vi "ORS_AlazarDLLAcq_Start.vi"(8 "error in (no error)":errorcluster, 11 "ATSHandle":u32) -> (0 "error out":errorcluster, 3 "ATSHandle_out":u32)   [LabVIEW 2024]
panel:
  out "path out":path
  out "return code":i32
  out "dt":u32=26
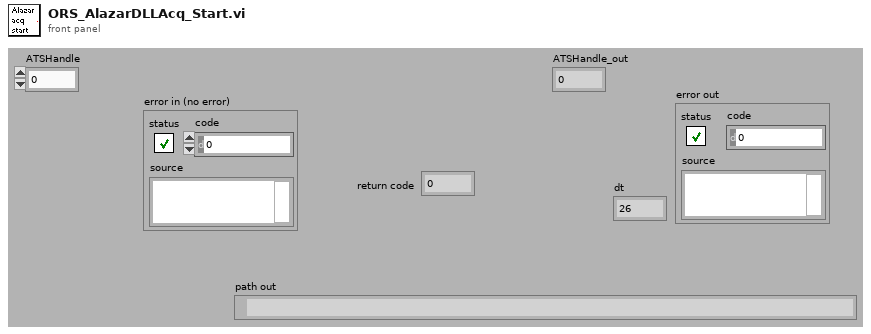
[diagram p1: front panel]
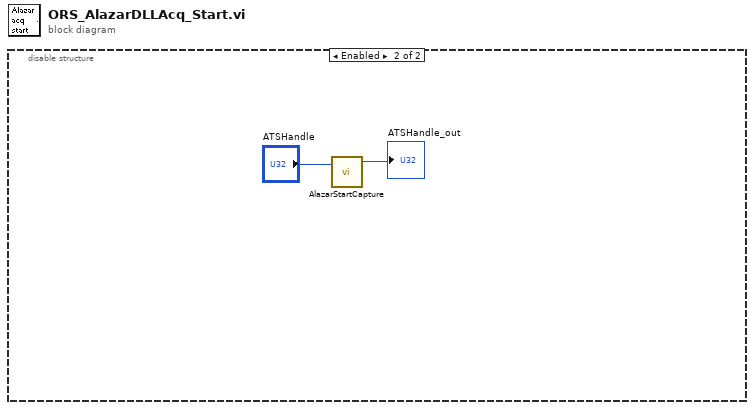
[diagram p0: block diagram]
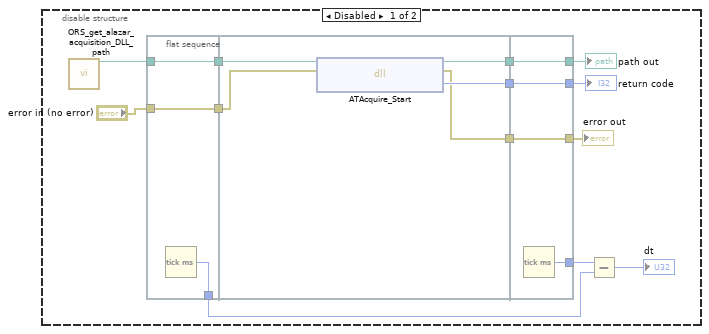
[diagram p2: hidden frame]
diagram:
  n1 = disable-structure shown="Enabled" {
    frame Disabled {
      n2 = call "ORS_get_alazar_acquisition_DLL_path.vi"() -> ("Alazar Acquisition DLL path"=w3:path)  [unwired: 10 in, 1 out]
      n3 = flat-sequence {
        tunnel: w3 -> [w16]
        tunnel: [w16] -> w13
        tunnel: [w15] -> w7
        tunnel: [w14] -> w12
        tunnel: "error in (no error)" -> [w14]
        tunnel: [w21] -> w11
        tunnel: w13 -> [w20]
        tunnel: [w19] -> w10
        tunnel: w12 -> [w18]
        tunnel: [w17] -> w9
        tunnel: [w25] -> w8
        tunnel: w11 -> [w25]
        tunnel: [w24] -> w6
        tunnel: [w23] -> w4
        tunnel: w10 -> [w23]
        tunnel: [w22] -> w1
        tunnel: w9 -> [w22]
        frame #0 {
          n4 = Tick Count (ms)() -> (millisecond timer value=w15:u32)
        }
        frame #1 {
          n5 = dll-call lib="Z:/Software/AlazarTech/ATS-SDK/5.6.3/ATS9462-SDK/Dual Port Async/C/PostBuffer_Recommended/at_acquire/Release/at_acquire.dll" fn="ATAcquire_Start" ("at_acquire.dll:TestFunc")(path in=w20, error in=w18) -> (path out=w19:path, error out=w17:errorcluster, "return type"=w21:i32)  [unwired: 1 in]
        }
        frame #2 {
          n6 = Tick Count (ms)() -> (millisecond timer value=w24:u32)
        }
      }
      n7 = Subtract(x=w6, y=w7) -> (x-y=→"dt":u32)
      "return code" <- w8
      "path out" <- w4
      "error out" <- w1
    }
    frame Enabled {
      n8 = call "AlazarStartCapture.vi"("Handle"="ATSHandle") -> ("Handle"=→"ATSHandle_out":u32)  [unwired: 1 in, 2 out]
    }
  }
